vi "局部旋转.vi"(10 "角度输入":dbl[](array[numeric]), 11 "取向输入":dbl[][](array[numeric])) -> (3 "取向输出":dbl[][](array[numeric]))   [LabVIEW 2017]
uses:
  <vilib>/Analysis/baseanly.llb/Real A x B.vi
  <vilib>/Analysis/Matrix/Numeric/Conversions/Matrix To Array - RM.vi
  <vilib>/Analysis/NI_AALBase.lvlib
  <vilib>/Analysis/Matrix/NI_Matrix.lvlib
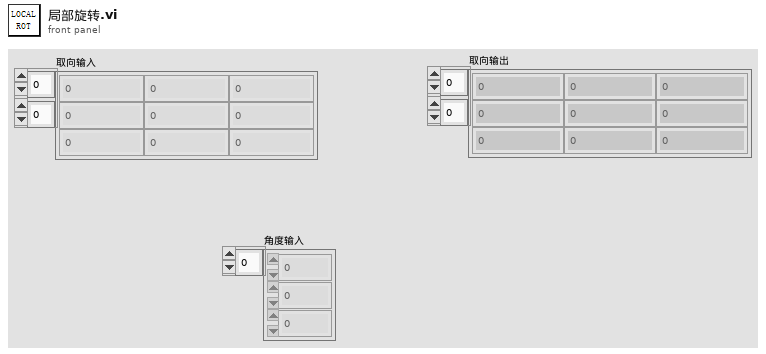
[diagram p1: front panel]
types:
  T1 = typedef "NI_Matrix.lvlib/RealMatrix.ctl" = dbl[][]
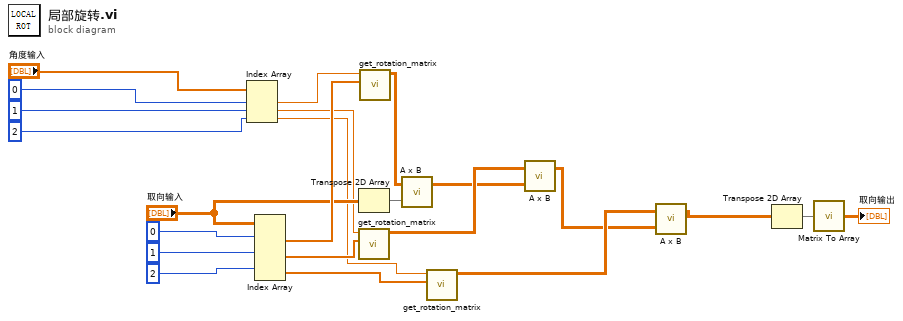
[diagram p0: block diagram]
diagram:
  n1 = Index Array(array="角度输入", index #1=0 ("index"), index #2=1 ("index"), index #3=2 ("index")) -> (element #1=w21:dbl, element #2=w10:dbl, element #3=w9:dbl)
  n2 = Index Array(array="取向输入", index (row) #1=0 ("index"), index (row) #2=1 ("index"), index (row) #3=2 ("index")) -> (element #1=w23:dbl[], element #2=w11:dbl[], element #3=w8:dbl[])  [unwired: 3 in]
  n3 = Transpose 2D Array(2D array="取向输入") -> (transposed array=w5:dbl[][])
  n4 = call "get_rotation_matrix.vi"("rotation_axis"=w11, "rotation_angle"=w10) -> ("rotation_matrix"=w4:dbl[][])  [unwired: 9 in]
  n5 = call "get_rotation_matrix.vi"("rotation_axis"=w23, "rotation_angle"=w21) -> ("rotation_matrix"=w6:dbl[][])  [unwired: 9 in]
  n6 = call-poly <vilib>:"A x B.vi"("B"=w5, "A"=w6) -> ("A x B"=w3:T1)  [unwired: 1 out]
  n7 = call "get_rotation_matrix.vi"("rotation_axis"=w8, "rotation_angle"=w9) -> ("rotation_matrix"=w2:dbl[][])  [unwired: 9 in]
  n8 = call-poly <vilib>:"A x B.vi"("B"=w3, "A"=w4) -> ("A x B"=w1:T1)  [unwired: 1 out]
  n9 = call-poly <vilib>:"A x B.vi"("B"=w1, "A"=w2) -> ("A x B"=w7:T1)  [unwired: 1 out]
  n10 = Transpose 2D Array(2D array=w7) -> (transposed array=w13:T1)
  n11 = call-poly <vilib>:"Matrix To Array.vi"("Real Matrix"=w13) -> ("Real 2D Array"=→"取向输出":dbl[][])
